vi "Post-Post-Build Action.vi"() -> ()   [LabVIEW 2020]
uses:
  <vilib>/Utility/miscctls.llb/LVMapReplaceAction.ctl
  <vilib>/Utility/traverseref.llb/TRef TravTarget.ctl
  dee71e12-324b-4db4-9417-184fb5b856f7.vi
  <vilib>/AppBuilder/AB_API_Simple/Get Build Specification Version (path).vi
  <vilib>/Utility/traverseref.llb/VI Scripting - Traverse.lvlib
  <vilib>/AppBuilder/AB_API_Simple/NI_App_Builder_API.lvlib
panel:
  out "Zipping...":path
  out "Deleting .vims from Library":path
  out "Deleting .vim from disk":path
  out "Scanning VI...":path
  in  "Folder Path (Empty: Source Distrubution Built Folder)":path
  # "Run this after the source distribution build - it cannot be run automatically as a post build step as it locks up the IDE"
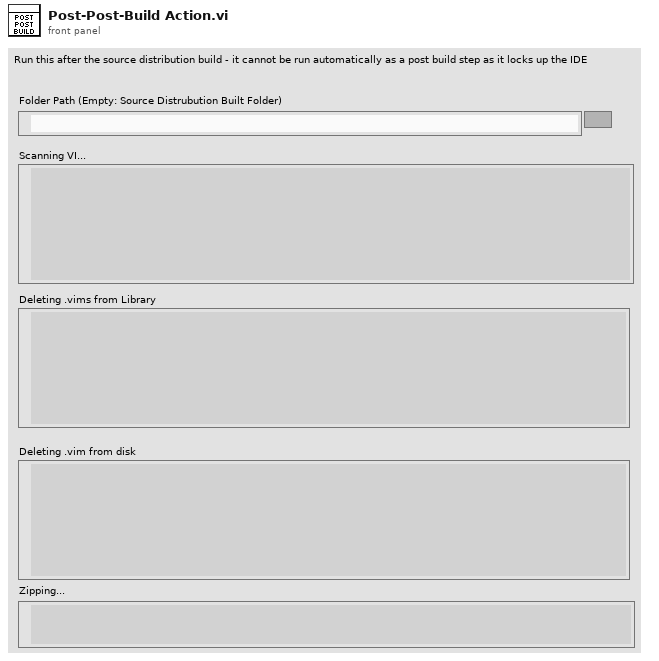
[diagram p1: front panel]
types:
  T1 = typedef "NI_App_Builder_API.lvlib/Build Specification Version.ctl" = cluster{"Major":u16, "Minor":u16, "Fix":u16, "Build":u16}
  T2 = typedef "LVMapReplaceAction.ctl" = enum32{"Modify Entry only if found", "Add or Modify Entry", "Delete Entry"}
  T3 = typedef "TRef TravTarget.ctl" = enum16{"FP", "BD", "Other"}
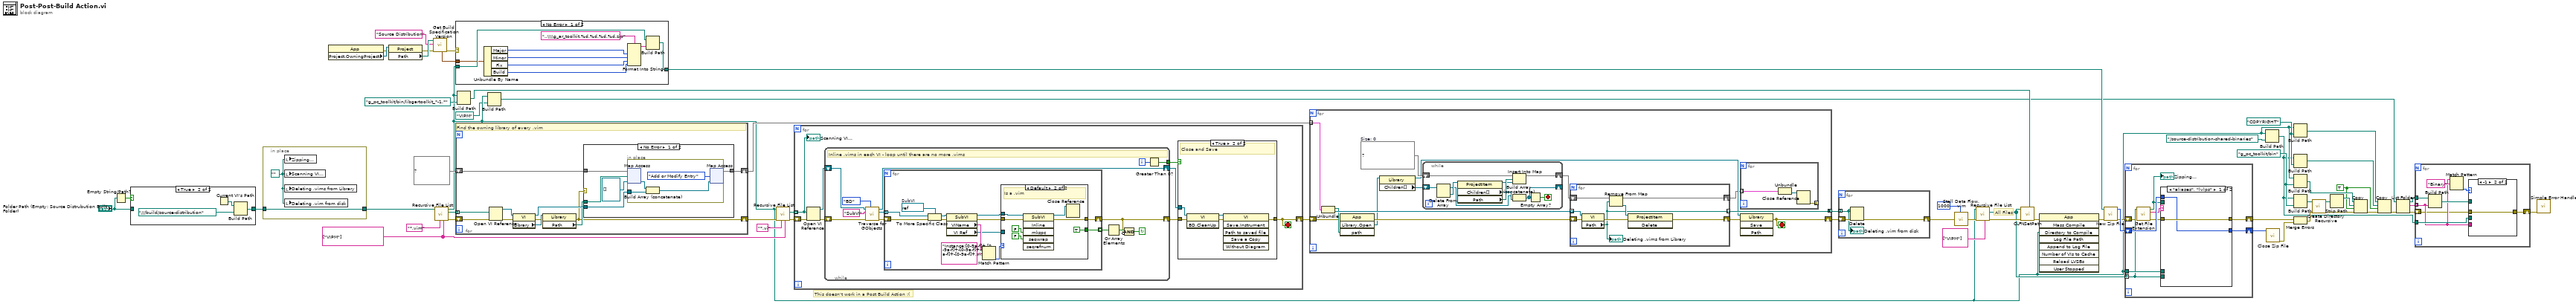
[diagram p0: block diagram]
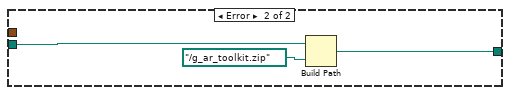
[diagram p2: hidden frame]
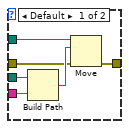
[diagram p3: hidden frame]
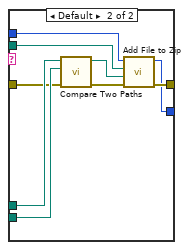
[diagram p4: hidden frame]
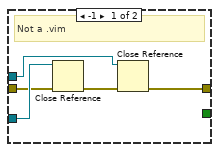
[diagram p6: hidden frame]
diagram:
  w17 = TRUE ("overwrite (F)")
  w25 = path "COPYRIGHT" ("name or relative path")
  w28 = path "g_pc_toolkit/bin" ("name or relative path")
  w34 = string[] ["VIPM"] ("Folders to Exclude")
  # "All Files"
  # "This doesn't work in a Post Build Action :("
  n1 = Empty String/Path?(string/path="Folder Path (Empty: Source Distrubution Built Folder)") -> (empty?=w49:bool)
  n2 = case shown="True" w49 {
    tunnel: [w63 w64] -> w48
    tunnel: "Folder Path (Empty: Source Distrubution Built Folder)" -> [w63 _]
    frame False {
    }
    frame True {
      n3 = Current VI's Path() -> (path=w66:path)
      n4 = Build Path(base path=w66, name or relative path=path "../../../build/source-distribution") -> (appended path=w64:path)
    }
  }
  n5 = in-place {
    in-place-border: [w68] -> w50
    in-place-border: w48 -> [w68]
    w67 = path "" ("Scanning VI...")
    n6 = local write "Zipping..."(w67) -> ()
    n7 = local write "Scanning VI..."(w67) -> ()
    n8 = local write "Deleting .vims from Library"(w67) -> ()
    n9 = local write "Deleting .vim from disk"(w67) -> ()
  }
  n10 = property class="App"() -> (error out=w1:errorcluster, "Project.OwningProject"=w7:refnum<vi>)  [unwired: 2 in, 1 out]
  n11 = property class="Project"(reference=w7, error in=w1) -> (error out=w2:errorcluster, "Path"=w6:path)  [unwired: 1 out]
  n12 = call-poly <vilib>:"Get Build Specification Version.vi"("error in (no error)"=w2, "Name of build specification"="Source Distribution", "Path to project"=w6) -> ("error out"=w3:errorcluster, "Build Specification Version"=w4:T1)  [unwired: 7 in]
  n13 = call <vilib>:"Recursive File List.vi"("Folders to Exclude"=w34, "pattern"="*.vim", "Folder Path"=w50) -> ("error out"=w60:errorcluster, "All Files in Dir"=w61:path[], "dup Folder Path"=w16:path)  [unwired: 4 in, 2 out]
  n14 = case shown="No Error" w3 {
    tunnel: [w77 w78] -> w46
    tunnel: w16 -> [w76 w80]
    tunnel: w4 -> [w75 _]
    frame No Error {
      n15 = Unbundle By Name(w75) -> ("Major"=w74:u16, "Minor"=w73:u16, "Fix"=w72:u16, "Build"=w71:u16)
      n16 = Format Into String(format string="..\\\\g_ar_toolkit.%d.%d.%d.%d.zip", w74, w73, w72, w71) -> (resulting string=w69:string)  [unwired: 2 in, 1 out]
      n17 = Build Path(base path=w76, name or relative path=w69) -> (appended path=w77:path)
    }
    frame Error {
      n18 = Build Path(base path=w80, name or relative path=path "../g_ar_toolkit.zip") -> (appended path=w78:path)
    }
  }
  n19 = for {
    tunnel: w61 -> [w88] mode=indexing
    shift-right: [w86] -> w53
    shift-left: map{path, refnum<vi>[]} {} ("Size: 0") -> [w85]
    shift-right: [w81] -> w58
    shift-left: w60 -> [w91]
    # "Find the owning library of every .vim"
    n20 = Open VI Reference(vi path=w88, error in (no error)=w91) -> (vi reference=w90:refnum<vi>, error out=w89:errorcluster)  [unwired: 4 in]
    n21 = property class="VI"(reference=w90, error in=w89) -> (reference out=w87:refnum<vi>, error out=w83:errorcluster, "Library"=w84:refnum<vi>)
    n22 = property class="Library"(reference=w84, error in=w83) -> (error out=w81:errorcluster, "Path"=w82:path)  [unwired: 1 out]
    n23 = case shown="No Error" w81 {
      tunnel: w87 -> [w96 _]
      tunnel: [w94 w101] -> w86
      tunnel: w85 -> [w93 w101]
      tunnel: w82 -> [w92 _]
      frame No Error {
        n24 = in-place {
          in-place-border: w96 -> [w98]
          n25 = in-place-map #1(w93, w92, refnum<vi>[] []) -> (w100:refnum<vi>[])  [unwired: 1 out]
          n26 = Build Array (concatenate)(w100, w98) -> (w97:refnum<vi>[])
          n27 = in-place-map #1(w97, LVMapReplaceAction."Add or Modify Entry" ("action")) -> (w94:map{path, refnum<vi>[]})  [unwired: 2 out]
        }
      }
      frame Error {
      }
    }
  }
  n28 = Build Path(base path=w16, name or relative path=path "g_pc_toolkit/bin/libgartoolkit_*-1.*") -> (appended path=w30:path)
  n29 = Build Path(base path=w16, name or relative path=path "VIPM") -> (appended path=w14:path)
  n30 = call <vilib>:"Recursive File List.vi"("Folders to Exclude"=w34, "pattern"="*.vi", "error in (no error)"=w58, "Folder Path"=w16) -> ("error out"=w56:errorcluster, "All Files in Dir"=w55:path[])  [unwired: 3 in, 3 out]
  n31 = for {
    shift-right: [w103] -> w54
    shift-left: w56 -> [w107]
    tunnel: w55 -> [w106] mode=indexing
    stop <- w103 stop-if-true
    n32 = Open VI Reference(vi path=w106, error in (no error)=w107) -> (vi reference=w108:refnum<vi>, error out=w102:errorcluster)  [unwired: 4 in]
    n33 = while {
      shift-right: [w120] -> w104
      shift-left: w108 -> [w121]
      shift-right: [w110] -> w109
      shift-left: w102 -> [w119]
      tunnel: [w113] -> w105
      i -> [w114]
      stop <- w111 continue-if-true
      # "Inline .vims in each VI - loop until there are no more .vims"
      n34 = call <vilib>:"Traverse for GObjects.vi"("Traverse Target"=TRef_TravTarget."BD", "error in (no error)"=w119, "Class Name"="SubVI", "VI Refnum"=w121) -> ("error out"=w118:errorcluster, "References"=w116:refnum<vi>[], "dup VI Refnum"=w120:refnum<vi>)  [unwired: 4 in, 1 out]
      n35 = for {
        shift-right: [w129] -> w110
        shift-left: w118 -> [w135]
        tunnel: w116 -> [w134] mode=indexing
        tunnel: [w128] -> w122 mode=indexing
        w133 = refnum<vi> refnum  # SubVI
        n36 = To More Specific Class(target class=w133, reference=w134, error in=w135) -> (specific class reference=w132:refnum<vi>, error out=w131:errorcluster)
        n37 = property class="SubVI"(reference=w132, error in=w131) -> (reference out=w124:refnum<vi>, error out=w127:errorcluster, "VIName"=w130:string, "VI Ref"=w125:refnum<vi>)
        n38 = Match Pattern(string=w130, regular expression="Instance:[0-9a-f]+-[0-9a-f]+-[0-9a-f]+-[0-9a-f]+-[0-9a-f]+.vi$") -> (offset past match=w126:i32)  [unwired: 1 in, 3 out]
        n39 = case shown="Default" w126 {
          tunnel: [w140 w147] -> w129
          tunnel: w125 -> [w138 _]
          tunnel: [_ TRUE] -> w128
          tunnel: w127 -> [w136 w142]
          tunnel: w124 -> [w139 w145]
          frame -1 {
            # "Not a .vim"
            n40 = Close Reference(reference=w138, error in (no error)=w136) -> (error out=w137:errorcluster)
            n41 = Close Reference(reference=w139, error in (no error)=w137) -> (error out=w140:errorcluster)
          }
          frame Default {
            # "Is a .vim"
            n42 = invoke class="SubVI" method="Inline"(reference=w145, error in=w142, "mkspc"=FALSE ("Make Space in Block Diagram"), "seqwrap"=FALSE ("Wrap in Sequence")) -> (reference out=w141:refnum<vi>, error out=w147:errorcluster)  [unwired: 2 in, 4 out]
            n43 = Close Reference(reference=w141) -> ()  [unwired: 1 in, 1 out]
          }
        }
      }
      n44 = Or Array Elements(Boolean array=w122) -> (logical OR=w115:bool)
      n45 = Compound Arithmetic op=AND(w115, invert w110) -> (w111:bool)
      n46 = Greater Than 0?(x=w114) -> (x > 0?=w113:bool)
    }
    n47 = case shown="True" w105 {
      tunnel: w104 -> [_ w153]
      tunnel: w109 -> [w148 w152]
      tunnel: [w148 w149] -> w103
      frame False {
        # "No Updates"
      }
      frame True {
        # "Close and Save"
        n48 = invoke class="VI" method="BD.CleanUp"(reference=w153, error in=w152) -> (reference out=w151:refnum<vi>, error out=w150:errorcluster)  [unwired: 1 in, 1 out]
        n49 = invoke class="VI" method="Save.Instrument"(reference=w151, error in=w150) -> (error out=w149:errorcluster)  [unwired: 4 in, 5 out]
      }
    }
    "Scanning VI..." <- w106
  }
  n50 = for {
    shift-right: [w154] -> w51
    shift-left: w54 -> [w163]
    tunnel: w53 -> [w167] mode=indexing
    tunnel: [w165] -> w52 mode=concatenating
    stop <- w154 stop-if-true
    w158 = map{path, refnum<vi>} {}  # Size: 0
    n51 = Unbundle(w167) -> ("Library"=w164:path, w166:refnum<vi>[])
    n52 = invoke class="App" method="Library.Open"(error in=w163, "path"=w164) -> (error out=w162:errorcluster, "Open Library"=w160:refnum<vi>)  [unwired: 2 in, 2 out]
    n53 = property class="Library"(reference=w160) -> (reference out=w156:refnum<vi>, "Children[]"=w159:refnum<vi>[])  [unwired: 1 in, 1 out]
    n54 = while {
      shift-right: [w172] -> _
      shift-left: w159 -> [w180]
      shift-right: [w174] -> w157
      shift-left: w158 -> [w173]
      stop <- w171 stop-if-true
      n55 = Delete From Array(array=w180) -> (deleted portion=w179:refnum<vi>, array with subset deleted=w177:refnum<vi>[])  [unwired: 2 in]
      n56 = property class="ProjectItem"(reference=w179) -> (reference out=w175:refnum<vi>, "Children[]"=w178:refnum<vi>[], "Path"=w176:path)  [unwired: 1 in, 1 out]
      n57 = Insert Into Map(map in=w173, key=w176, value=w175) -> (map out=w174:map{path, refnum<vi>})  [unwired: 2 out]
      n58 = Build Array (concatenate)(w177, w178) -> (w172:refnum<vi>[])
      n59 = Empty Array?(array=w172) -> (empty?=w171:bool)
    }
    n60 = for {
      shift-right: [w183] -> w161
      shift-left: w162 -> [w186]
      tunnel: w166 -> [w185] mode=indexing
      tunnel: [w182] -> w165 mode=indexing
      shift-right: [w181] -> w155
      shift-left: w157 -> [w188]
      n61 = property class="VI"(reference=w185, error in=w186) -> (error out=w184:errorcluster, "Path"=w182:path)  [unwired: 1 out]
      "Deleting .vims from Library" <- w182
      n62 = Remove From Map(10:w182, 11:w188) -> (1:w187:refnum<vi>, 3:w181:map{path, refnum<vi>})  [unwired: 1 out]
      n63 = invoke class="ProjectItem" method="Delete"(reference=w187, error in=w184) -> (error out=w183:errorcluster)  [unwired: 1 in, 2 out]
    }
    n64 = for {
      tunnel: w155 -> [w170] mode=indexing
      tunnel: [w168] -> _ mode=indexing
      n65 = Unbundle(w170) -> (w169:refnum<vi>)  [unwired: 1 out]
      n66 = Close Reference(reference=w169) -> (error out=w168:errorcluster)  [unwired: 1 in]
    }
    n67 = invoke class="Library" method="Save"(reference=w156, error in=w161) -> (error out=w154:errorcluster)  [unwired: 2 in, 3 out]
  }
  n68 = for {
    tunnel: w52 -> [w189] mode=indexing
    shift-right: [w190] -> w38
    shift-left: w51 -> [w191]
    n69 = Delete(path (use dialog)=w189, error in=w191) -> (error out=w190:errorcluster)  [unwired: 3 in, 2 out]
    "Deleting .vim from disk" <- w189
  }
  n70 = call "Stall Data Flow.vim"("value in"=w38, "milliseconds to wait"=u32 1000) -> ("value out"=w36:errorcluster)  [unwired: 1 out]
  n71 = call <vilib>:"Recursive File List.vi"("Folders to Exclude"=string[] ["VIPM"], "error in (no error)"=w36, "Folder Path"=w16) -> ("error out"=w37:errorcluster, "All Files in Dir"=w32:path[])  [unwired: 4 in, 3 out]
  n72 = call "CLFNSetPath.vi"("New Path"=w30, "error in (no error)"=w37, "Files"=w32) -> ("error out"=w39:errorcluster)  [unwired: 7 in, 1 out]
  n73 = invoke class="App" method="Mass Compile"(error in=w39, "Directory to Compile"=w16) -> (error out=w40:errorcluster)  [unwired: 7 in, 8 out]
  n74 = call <vilib>:"New Zip File.vi"("error in (no error)"=w40, "target"=w46) -> ("error out"=w44:errorcluster, "zip file out"=w45:i64)  [unwired: 3 in, 1 out]
  n75 = for {
    shift-right: [w198] -> w43
    shift-left: w45 -> [w200]
    shift-right: [w199] -> w42
    shift-left: w44 -> [w195]
    tunnel: w32 -> [w196] mode=indexing
    tunnel: w16 -> [w197]
    n76 = call <vilib>:"Get File Extension.vi"("error in (no error)"=w195, "file"=w196) -> ("error out"=w194:errorcluster, "lowercase file extension"=w192:string, "dup file"=w193:path)  [unwired: 5 in, 2 out]
    "Zipping..." <- w193
    n77 = case shown="\"aliases\", \"lvlps\"" w192 {
      tunnel: w200 -> [w201 w210]
      tunnel: [w202 w208] -> w199
      tunnel: [w201 w207] -> w198
      tunnel: w197 -> [_ w206]
      tunnel: w196 -> [_ w205]
      tunnel: w193 -> [_ w204]
      tunnel: w194 -> [w202 w203]
      frame "aliases", "lvlps" {
      }
      frame Default {
        n78 = call <vilib>:"Compare Two Paths.vi"("error in (no error)"=w203, "Path 2"=w205, "Path 1"=w206) -> ("error out"=w209:errorcluster, "Relative Path from 1 to 2"=w211:path)  [unwired: 5 in, 2 out]
        n79 = call <vilib>:"Add File to Zip.vi"("error in (no error)"=w209, "destination path in zip"=w211, "source file path"=w204, "zip file in"=w210) -> ("error out"=w208:errorcluster, "zip file out"=w207:i64)  [unwired: 6 in]
      }
    }
  }
  n80 = Build Path(base path=w16, name or relative path=path "../source-distribution-shared-binaries") -> (appended path=w12:path)
  n81 = call <vilib>:"Close Zip File.vi"("zip file in"=w43) -> ("error out"=w41:errorcluster)  [unwired: 6 in]
  n82 = Build Path(base path=w16, name or relative path=w25) -> (appended path=w26:path)
  n83 = Build Path(base path=w12, name or relative path=w25) -> (appended path=w24:path)
  n84 = Build Path(base path=w16, name or relative path=w28) -> (appended path=w21:path)
  n85 = Build Path(base path=w12, name or relative path=w28) -> (appended path=w20:path)
  n86 = Merge Errors(w42, w41) -> (w23:errorcluster)
  n87 = call <vilib>:"Create Directory Recursive.vi"("error in (no error)"=w23, "directory"=w20) -> ("error out"=w22:errorcluster, "directory copy"=w19:path)  [unwired: 3 in, 1 out]
  n88 = Strip Path(path=w19) -> (stripped path=w18:path)  [unwired: 1 out]
  n89 = Copy(8:w22, 9:w17, 10:w18, 11:w21) -> (0:w27:errorcluster)  [unwired: 1 in, 2 out]
  n90 = Copy(8:w27, 9:w17, 10:w24, 11:w26) -> (0:w9:errorcluster)  [unwired: 1 in, 2 out]
  n91 = List Folder(path=w14, error in=w9) -> (path out=w13:path, filenames=w8:string[], error out=w10:errorcluster)  [unwired: 2 in, 1 out]
  n92 = for {
    tunnel: w13 -> [w219]
    tunnel: w8 -> [w214] mode=indexing
    tunnel: w12 -> [w215]
    shift-right: [w212] -> w11
    shift-left: w10 -> [w213]
    n93 = Build Path(base path=w219, name or relative path=w214) -> (appended path=w216:path)
    n94 = Match Pattern(string=w214, regular expression="Binary") -> (offset past match=w217:i32)  [unwired: 1 in, 3 out]
    n95 = case shown="-1" w217 {
      tunnel: w216 -> [w225 _]
      tunnel: w215 -> [w224 _]
      tunnel: w214 -> [w223 _]
      tunnel: w213 -> [w221 w226]
      tunnel: [w220 w226] -> w212
      frame Default {
        n96 = Build Path(base path=w224, name or relative path=w223) -> (appended path=w222:path)
        n97 = Move(source path=w225, error in=w221, 10:w222) -> (error out=w220:errorcluster)  [unwired: 2 in, 2 out]
      }
      frame -1 {
      }
    }
  }
  n98 = call <vilib>:"Simple Error Handler.vi"("error in (no error)"=w11) -> ()  [unwired: 4 in, 5 out]
